vi "Serial Com Logger.vi"(7 "Action":T1(ring), 8 "error in":errorcluster, 9 "Buffer(lines)":i32=5000, 10 "Log File":path, 11 "Input String":string) -> (0 "error out":errorcluster, 3 "Log":string)   [LabVIEW 2018]
uses:
  Main/Main Globals.vi
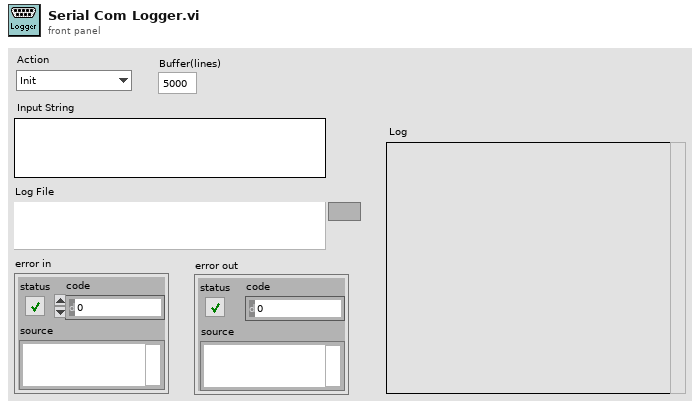
[diagram p1: front panel]
types:
  T1 = enum16{"Init", "Reset", "Read", "Update", "Close"}
  T2 = enum16{"open", "replace", "create", "open or create", "replace or create", "replace or create with confirmation"}
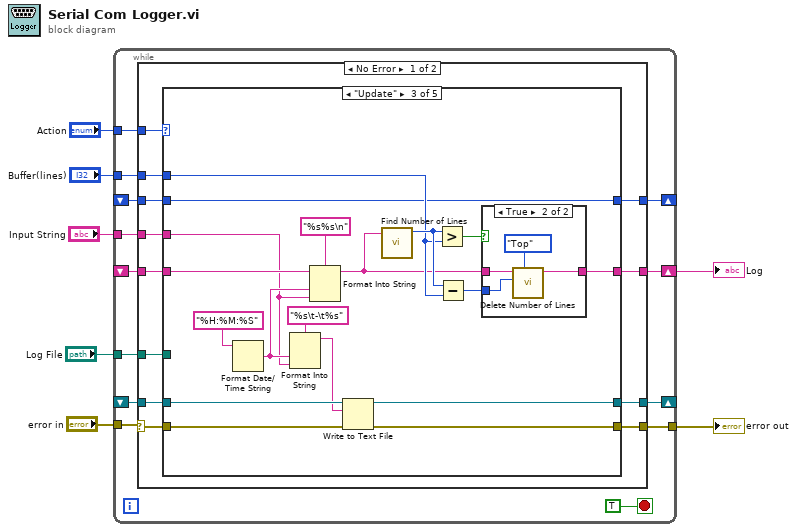
[diagram p0: block diagram]
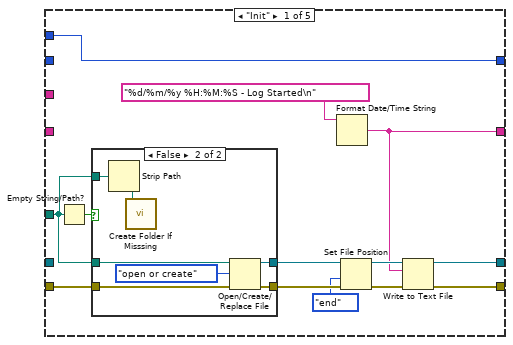
[diagram p2: hidden frame]
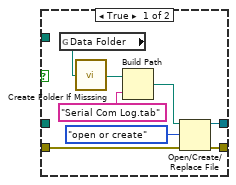
[diagram p3: hidden frame]
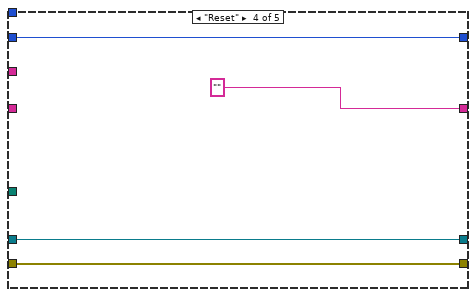
[diagram p6: hidden frame]
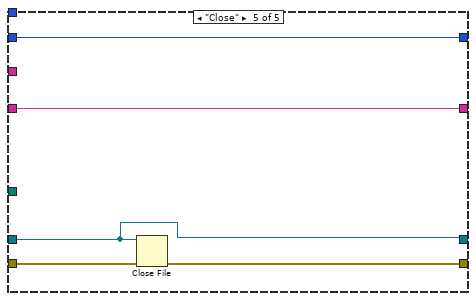
[diagram p7: hidden frame]
diagram:
  n1 = while {
    tunnel: "error in" -> [w19]
    tunnel: [w15] -> w6
    tunnel: "Action" -> [w18]
    tunnel: "Log File" -> [w17]
    tunnel: "Input String" -> [w16]
    shift-right: [w14] -> _
    shift-left: _ -> [w13]
    shift-right: [w12] -> w1
    shift-left: _ -> [w11]
    tunnel: "Buffer(lines)" -> [w10]
    shift-right: [w9] -> _
    shift-left: _ -> [w8]
    stop <- TRUE stop-if-true
    n2 = case shown="No Error" w19 {
      selector: w19 -> [w32 w99]
      tunnel: w18 -> [w31 _]
      tunnel: w17 -> [w30 _]
      tunnel: w16 -> [w29 _]
      tunnel: [w28 w99] -> w15
      tunnel: [w27 w100] -> w14
      tunnel: w13 -> [w26 w100]
      tunnel: [w25 w98] -> w12
      tunnel: w11 -> [w24 w98]
      tunnel: w10 -> [w23 _]
      tunnel: [w22 w97] -> w9
      tunnel: w8 -> [w21 w97]
      frame No Error {
        n3 = case shown="\"Update\"" w31 {
          tunnel: w32 -> [w44 w63 w82 w89 w95]
          tunnel: w30 -> [w43 _ _ _ _]
          tunnel: w29 -> [_ _ w65 _ _]
          tunnel: [w37 w63 w68 w89 w94] -> w28
          tunnel: [w36 w62 w69 w90 w93] -> w27
          tunnel: w26 -> [_ w62 w79 w90 w93]
          tunnel: [w34 w64 w71 "" ("Resulting String") w96] -> w25
          tunnel: w24 -> [_ w64 w77 _ w96]
          tunnel: w23 -> [w33 _ w74 _ _]
          tunnel: [w33 w61 w67 w88 w92] -> w22
          tunnel: w21 -> [_ w61 w67 w88 w92]
          frame "Init" {
            n4 = Empty String/Path?(string/path=w43) -> (empty?=w45:bool)
            n5 = case shown="False" w45 {
              tunnel: w44 -> [w48 w59]
              tunnel: [w47 w58] -> w42
              tunnel: w43 -> [_ w56]
              tunnel: w43 -> [_ w55]
              tunnel: [w46 w54] -> w41
              frame True {
                n6 = global read "Main Globals.vi" "Data Folder"() -> (w53:path)
                n7 = call "Create Folder If Misssing.vi"("Path In"=w53) -> ("Path Out"=w52:path)
                n8 = Build Path(base path=w52, name or relative path="Serial Com Log.tab") -> (appended path=w50:path)
                n9 = Open/Create/Replace File(file path (use dialog)=w50, error in=w48, operation (0:open)=T2."open or create") -> (refnum out=w46:refnum<file>, error out=w47:errorcluster)  [unwired: 3 in, 1 out]
              }
              frame False {
                n10 = Strip Path(path=w56) -> (stripped path=w57:path)  [unwired: 1 out]
                n11 = call "Create Folder If Misssing.vi"("Path In"=w57) -> ()  [unwired: 1 out]
                n12 = Open/Create/Replace File(file path (use dialog)=w55, error in=w59, operation (0:open)=T2."open or create") -> (refnum out=w54:refnum<file>, error out=w58:errorcluster)  [unwired: 3 in, 1 out]
              }
            }
            n13 = Format Date/Time String(time format string (%c)="%d/%m/%y %H:%M:%S - Log Started\n") -> (date/time string=w34:string)  [unwired: 2 in]
            n14 = Set File Position(refnum=w41, from (0:start)=enum16{"start", "end", "current"}."end", error in=w42) -> (refnum out=w39:refnum<file>, error out=w35:errorcluster)  [unwired: 1 in]
            n15 = Write to Text File(file (use dialog)=w39, text=w34, error in=w35) -> (refnum out=w36:refnum<file>, error out=w37:errorcluster)  [unwired: 1 in, 1 out]
          }
          frame "Read" {
          }
          frame "Update" {
            n16 = Format Date/Time String(time format string (%c)="%H:%M:%S") -> (date/time string=w66:string)  [unwired: 2 in]
            n17 = Format Into String(format string="%s\t-\t%s", w66, w65) -> (resulting string=w78:string)  [unwired: 2 in, 1 out]
            n18 = Format Into String(format string="%s%s\n", initial string=w77, w66, w65) -> (resulting string=w72:string)  [unwired: 1 in, 1 out]
            n19 = Write to Text File(file (use dialog)=w79, text=w78, error in=w82) -> (refnum out=w69:refnum<file>, error out=w68:errorcluster)  [unwired: 1 in, 1 out]
            n20 = call "Find Number of Lines.vi"("String"=w72) -> ("Number of Lines"=w75:i32)  [unwired: 10 in]
            n21 = Greater?(x=w75, y=w74) -> (0:w76:bool)
            n22 = Subtract(x=w75, y=w74) -> (x-y=w73:i32)
            n23 = case shown="True" w76 {
              tunnel: w73 -> [_ w86]
              tunnel: w72 -> [w83 w87]
              tunnel: [w83 w85] -> w71
              frame False {
              }
              frame True {
                n24 = call "Delete Number of Lines.vi"("Position"=enum16{"Top", "Bottom", "Line N"}."Top", "Number of Lines"=w86, "String"=w87) -> ("Resulting String"=w85:string)  [unwired: 8 in]
              }
            }
          }
          frame "Reset" {
          }
          frame "Close" {
            n25 = Close File(refnum=w93, error in=w95) -> (error out=w94:errorcluster)  [unwired: 1 out]
          }
        }
      }
      frame Error {
      }
    }
  }
  "error out" <- w6
  "Log" <- w1
